vi "ParseOutputs.vi"(8 "error in (no error)":errorcluster, 9 "test details":string, 10 "successful?":bool, 11 "RunTests in":refnum<class "RunVITester.lvclass">) -> (0 "error out":errorcluster, 1 "Output/Failure":string, 2 "CLI Process Return Code":i32, 3 "RunTests out":refnum<class "RunVITester.lvclass">)   [LabVIEW 2015, in "RunVITester.lvclass"]
uses:
  RunVITester.lvclass
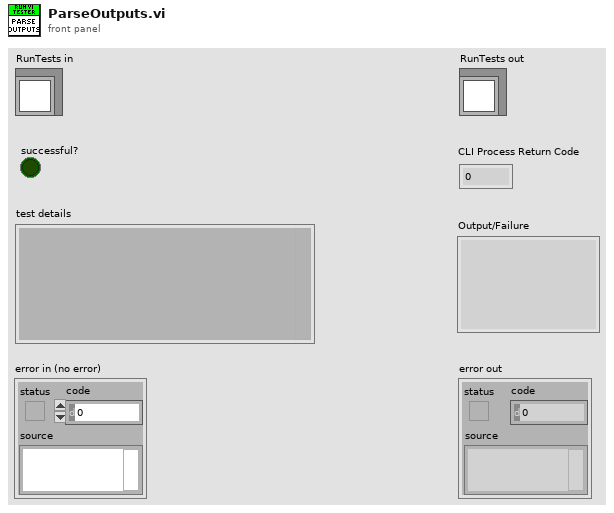
[diagram p1: front panel]
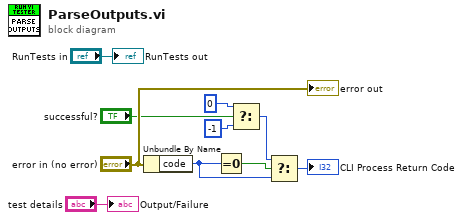
[diagram p0: block diagram]
diagram:
  n1 = Unbundle By Name("error in (no error)") -> ("code"=w7:i32)
  n2 = Equal To 0?(x=w7) -> (x = 0?=w8:bool)
  n3 = Select(t=0 ("code"), s="successful?", f=-1 ("code")) -> (s? t:f=w3:i32)
  n4 = Select(t=w3, s=w8, f=w7) -> (s? t:f=→"CLI Process Return Code":i32)
  "error out" <- "error in (no error)"
  "RunTests out" <- "RunTests in"
  "Output/Failure" <- "test details"
